vi "Load Logging Config File.vi"(0 "Logging Config File Location":path, 2 "error in":errorcluster) -> (3 "IP Address":string, 4 "Descriptions":string[](array[string]), 5 "S7 Read Write Array":T1[](array[typedef]) {"Address Areas" items=["I/O (P)"=128, "Input (I)"=129, "Output (Q)"=130, "Bit Memory (M)"=131, "Data (DB)"=132, "Instance Data (DI)"=133, "Local Data (L)"=134, "Predecessor Local Data (VL)"=135]; "Read / Write" items=["Read"=4, "Write"=5]; "Bit Number / Byte Length" max=7 step=1}, 6 "error out":errorcluster)   [LabVIEW 2017]
uses:
  S7 Read Write Cluster.ctl
  Data Type.ctl
  S7 TCP.lvlib
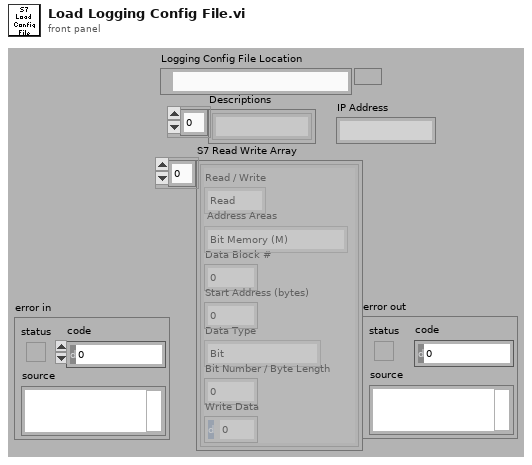
[diagram p1: front panel]
types:
  T1 = typedef "S7 TCP.lvlib/S7 Read Write Cluster.ctl" = cluster{"Read / Write":u8, "Address Areas":u8, "Data Block #":u16, "Start Address (bytes)":u32, "Data Type":T2, "Bit Number / Byte Length":u8, "Write Data":dbl}
  T2 = typedef "S7 TCP.lvlib/Data Type.ctl" = enum16{"Bit", "Byte (U8)", "Signed Byte (I8)", "Word (U16)", "Signed Word (I16)", "Long (U32)", "Signed Long (I32)", "Real (SGL)", "Defined Byte Length"}
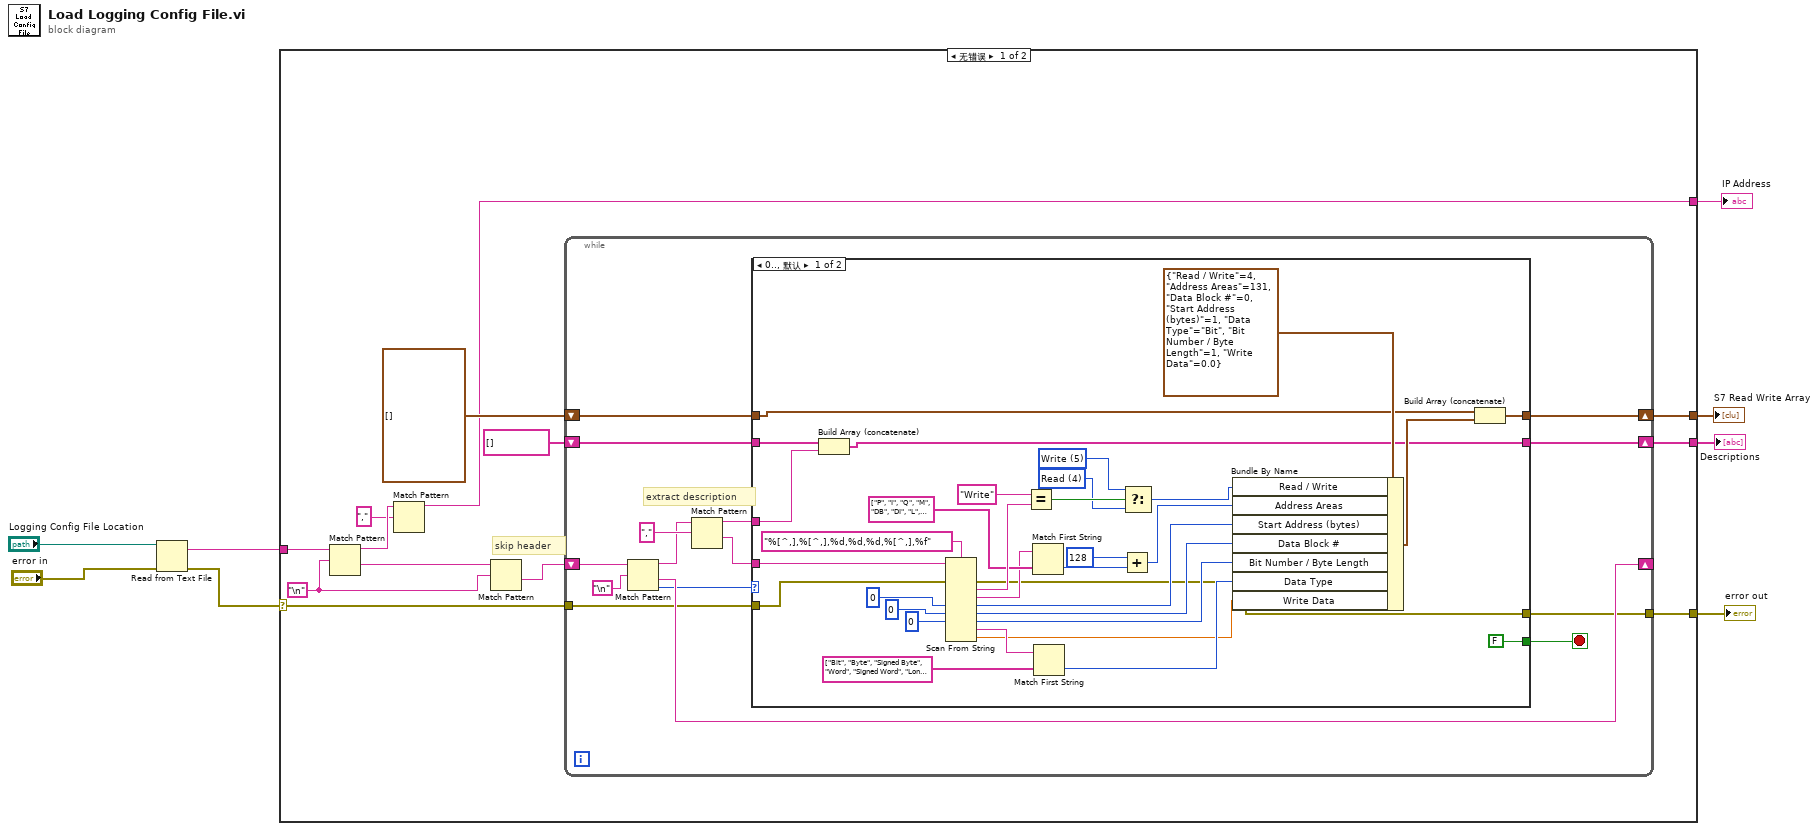
[diagram p0: block diagram]
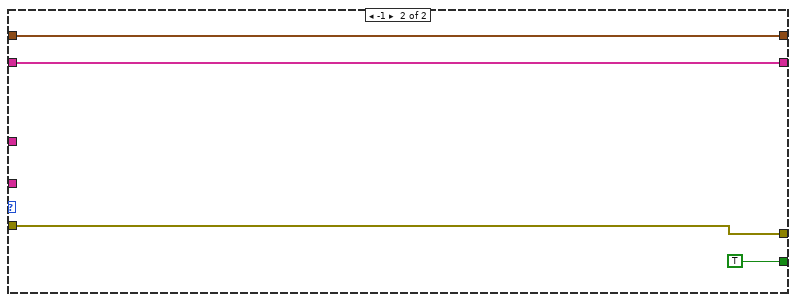
[diagram p2: hidden frame]
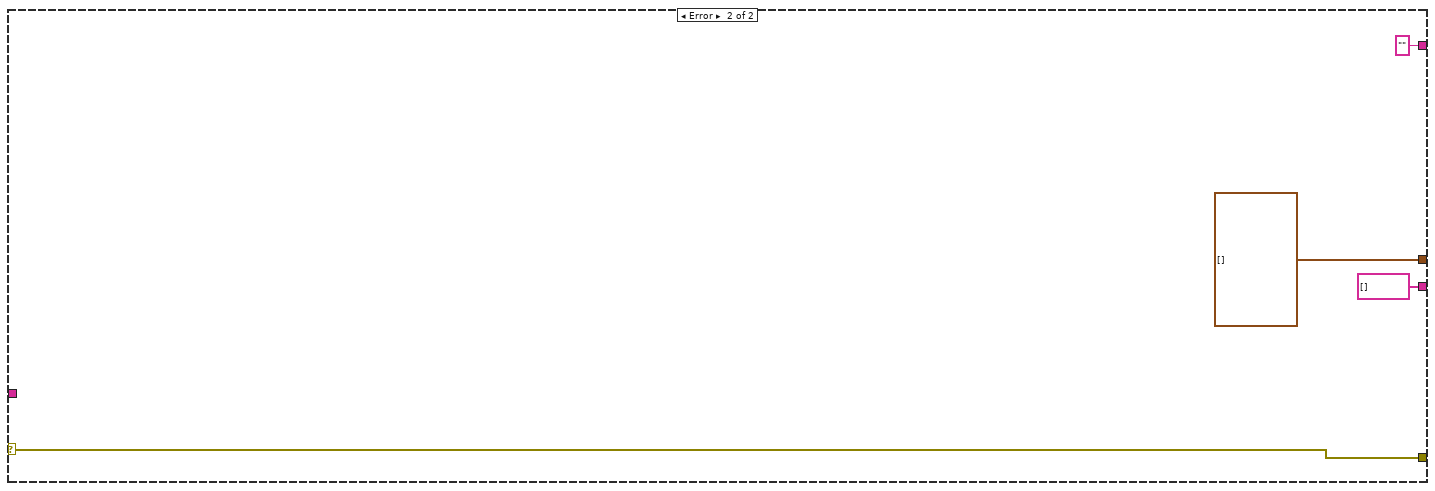
[diagram p3: hidden frame]
diagram:
  n1 = Read from Text File(file (use dialog)="Logging Config File Location", error in="error in") -> (text=w7:string, error out=w1:errorcluster)  [unwired: 4 out]
  n2 = case shown="无错误" w1 {
    selector: w1 -> [w12 w74]
    tunnel: w7 -> [w21 _]
    tunnel: [w20 T1[] []] -> w6
    tunnel: [w17 string[] [] ("Strings []")] -> w5
    tunnel: [w16 w74] -> w4
    tunnel: [w9 ""] -> w2
    frame No Error {
      w13 = "\n"
      # "skip header"
      n3 = Match Pattern(string=w21, regular expression=w13) -> (before substring=w11:string, after substring=w15:string)  [unwired: 3 out]
      n4 = Match Pattern(string=w11, regular expression=",") -> (before substring=w9:string)  [unwired: 4 out]
      n5 = Match Pattern(string=w15, regular expression=w13) -> (after substring=w14:string)  [unwired: 4 out]
      n6 = while {
        shift-right: [w34] -> _
        shift-left: w14 -> [w35]
        shift-right: [w31] -> w20
        shift-left: T1[] [] -> [w30]
        shift-right: [w24] -> w17
        shift-left: string[] [] ("Strings []") -> [w26]
        tunnel: w12 -> [w23]
        tunnel: [w22] -> w16
        stop <- w32 stop-if-true
        # "extract description"
        n7 = Match Pattern(string=w35, regular expression="\n") -> (before substring=w28:string, after substring=w34:string, offset past match=w33:i32)  [unwired: 2 out]
        n8 = Match Pattern(string=w28, regular expression=",") -> (before substring=w25:string, after substring=w27:string)  [unwired: 3 out]
        n9 = case shown="0.., 默认" w33 {
          tunnel: w27 -> [w67 _]
          tunnel: [FALSE TRUE] -> w32
          tunnel: [w42 w72] -> w31
          tunnel: w30 -> [w47 w72]
          tunnel: w26 -> [w41 w71]
          tunnel: w25 -> [w40 _]
          tunnel: [w39 w71] -> w24
          tunnel: w23 -> [w38 w70]
          tunnel: [w37 w70] -> w22
          frame 0.., Default {
            w58 = u8 4 items=["Read"=4, "Write"=5] ("Read / Write")
            w59 = u8 5 items=["Read"=4, "Write"=5] ("Read / Write")
            n10 = Build Array (concatenate)(w41, w40) -> (w39:string[])
            n11 = Scan From String(format string="%[^,],%[^,],%d,%d,%d,%[^,],%f", input string=w67, error in=w38, default 3=u32 0 ("Start Address (bytes)"), default 4=u16 0 ("Data Block #"), default 5=u8 0 ("Bit Number")) -> (error out=w37:errorcluster, output 1=w62:string, output 2=w55:string, output 3=w43:u32, output 4=w53:u16, output 5=w52:u8, output 6=w51:string, output 7=w48:dbl)  [unwired: 1 in, 6 out]
            n12 = Equal?(x="Write", y=w62) -> (x = y?=w60:bool)
            n13 = Match First String(2:string[] ["P", "I", "Q", "M", "DB", "DI", "L", "VL"] ("Strings []"), 3:w55) -> (0:w45:i32)  [unwired: 1 out]
            n14 = Match First String(2:string[] ["Bit", "Byte", "Signed Byte", "Word", "Signed Word", "Long", "Signed Long", "Real"] ("Strings []"), 3:w51) -> (0:w49:i32)  [unwired: 1 out]
            n15 = Add(x=u8 128 ("y"), y=w45) -> (x+y=w44:i32)
            n16 = Select(t=w59, s=w60, f=w58) -> (s? t:f=w57:u8)
            n17 = Bundle By Name(cluster=T1 {"Read / Write"=4, "Address Areas"=131, "Data Block #"=0, "Start Address (bytes)"=1, "Data Type"=enum."Bit", "Bit Number / Byte Length"=1, "Write Data"=0.0} ("MPI Read Cluster"), "Read / Write"=w57, "Address Areas"=w44, "Start Address (bytes)"=w43, "Data Block #"=w53, "Bit Number / Byte Length"=w52, "Data Type"=w49, "Write Data"=w48) -> (w46:T1)
            n18 = Build Array (concatenate)(w47, w46) -> (w42:T1[])
          }
          frame -1 {
          }
        }
      }
    }
    frame Error {
    }
  }
  "S7 Read Write Array" <- w6
  "Descriptions" <- w5
  "error out" <- w4
  "IP Address" <- w2
